vi "AlliGator Build Phasor Calibration Series.vi"(8 "Error In":errorcluster, 9 "Calibration Lifetime":dbl[unit]=1e-09, 10 "Phasor Frequency":dbl[unit]=80000000.0, 11 "Uncalibrated Phasor Series":T2[](array[typedef])) -> (0 "Error Out":errorcluster, 3 "Phasor Reference Series":T1={"m Array"=[], "phi Array"=[], "Phasor Frequency"=80000000.0, "Calibration Lifetime"=1e-09})   [LabVIEW 2021, in "AlliGator Phasor Calibration.lvlib"]
doc: "Packages the provided <B>Uncalibrated Phasor Series</b> as a <B>Phasor Reference Series</B>."
uses:
  Phasor/Phasor (g, s).ctl
  Phasor/Phasor Reference Series.ctl
  AlliGator Phasor Calibration.lvlib
  Phasor/Phasor.lvlib
  Utilities/Utilities.lvlib
panel:
  # "see the AlliGator License on the block diagram (Ctrl+E or Window:Show Block Diagram)"
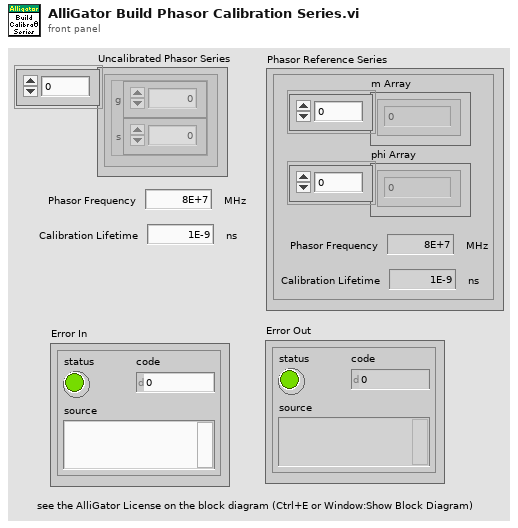
[diagram p1: front panel]
types:
  T1 = typedef "Phasor.lvlib/Phasor Reference Series.ctl" = cluster{"m Array":dbl[], "phi Array":dbl[], "Phasor Frequency":dbl[unit], "Calibration Lifetime":dbl[unit]}
  T2 = typedef "Phasor.lvlib/Phasor (g, s).ctl" = cluster{"g":dbl, "s":dbl}
  T3 = typedef "Phasor.lvlib/Phasor (m, phi).ctl" = cluster{"m":dbl, "phi":dbl}
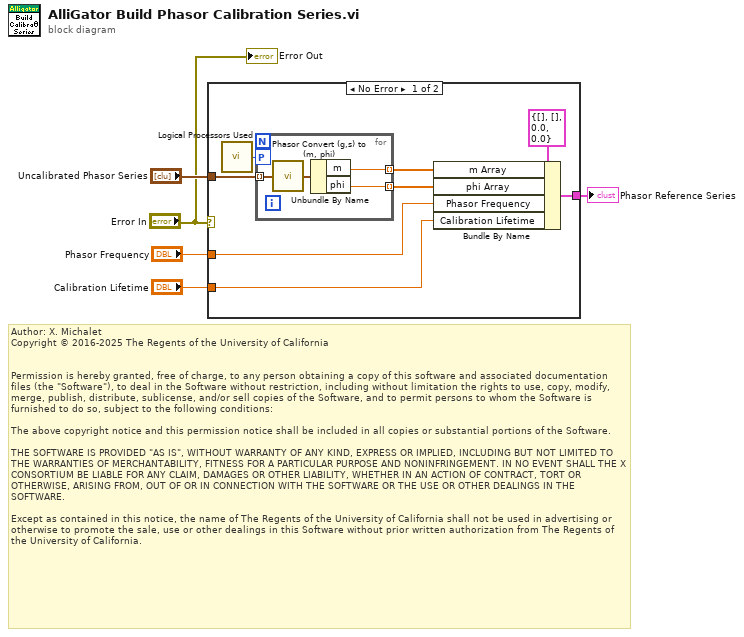
[diagram p0: block diagram]
diagram:
  # "Author: X. Michalet\nCopyright © 2016-2025 The Regents of the University of California\n \n\nPermission is hereby granted, free of charge, to any person obtaining a copy of this software and associated documentation files (the \"Software\"), to deal in the Software without restriction, including without limitation the rights to use, copy, modify, merge, publish, distribute, sublicense, and/or sell copies of the Software, and to permit persons to whom the Software is furnished to do so, subject to the following conditions:\n\nThe above copyright notice and this permission notice shall be included in all copies or substantial portions of the Software.\n\nTHE SOFTWARE IS PROVIDED \"AS IS\", WITHOUT WARRANTY OF ANY KIND, EXPRESS OR IMPLIED, INCLUDING BUT NOT LIMITED TO THE WARRANTIES OF MERCHANTABILITY, FITNESS FOR A PARTICULAR PURPOSE AND NONINFRINGEMENT. IN NO EVENT SHALL THE X CONSORTIUM BE LIABLE FOR ANY CLAIM, DAMAGES OR OTHER LIABILITY, WHETHER IN AN ACTION OF CONTRACT, TORT OR OTHERWISE, ARISING FROM, OUT OF OR IN CONNECTION WITH THE SOFTWARE OR THE USE OR OTHER DEALINGS IN THE SOFTWARE.\n\nExcept as contained in this notice, the name of The Regents of the University of California shall not be used in advertising or otherwise to promote the sale, use or other dealings in this Software without prior written authorization from The Regents of the University of California."
  n1 = case shown="No Error" "Error In" {
    tunnel: "Phasor Frequency" -> [w12 _]
    tunnel: "Calibration Lifetime" -> [w11 _]
    tunnel: [w10 _] -> w3
    tunnel: "Uncalibrated Phasor Series" -> [w9 _]
    frame No Error {
      n2 = call "Logical Processors Used.vi"() -> ("# Logical Processor Used"=w6:i32)  [unwired: 6 in]
      n3 = for {
        tunnel: w9 -> [w17] mode=indexing
        tunnel: [w16] -> w8 mode=indexing
        tunnel: [w15] -> w7 mode=indexing
        workers-P: w6 -> [_]
        n4 = call "Phasor Convert (g,s) to (m, phi).vi"("Phasor (g, s)"=w17) -> ("Phasor (m, phi)"=w14:T3)  [unwired: 8 in]
        n5 = Unbundle By Name(w14) -> ("m"=w16:dbl, "phi"=w15:dbl)
      }
      n6 = Bundle By Name(cluster=T1 {"m Array"=[], "phi Array"=[], "Phasor Frequency"=0.0, "Calibration Lifetime"=0.0} ("Phasor Reference Plot"), "m Array"=w8, "phi Array"=w7, "Phasor Frequency"=w12, "Calibration Lifetime"=w11) -> (w10:T1)
    }
    frame Error {
    }
  }
  "Phasor Reference Series" <- w3
  "Error Out" <- "Error In"
